vi "Last Ack Event.vi"(10 "Event":refnum<class "Event.lvclass">, 11 "Base Queue in":refnum<class "Base Queue.lvclass">) -> (3 "Base Queue out":refnum<class "Base Queue.lvclass">)   [LabVIEW 2021, in "jettl.lvlib" / "Base Queue.lvlib" / "Base Queue.lvclass"]
uses:
  Base Queue.lvclass
  Event/Event.lvclass
  Base Queue.lvclass/Base Queue.ctl
  Queue Mailbox/Queue Mailbox.lvlib
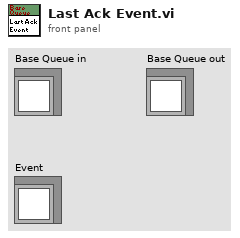
[diagram p1: front panel]
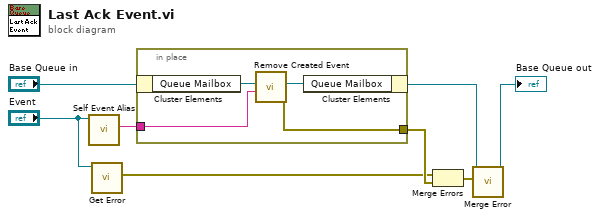
[diagram p0: block diagram]
diagram:
  n1 = call-dynamic "Self Event Alias.vi"("Event in"="Event") -> ("Self Event Alias"=w5:string)  [unwired: 10 in]
  n2 = call-dynamic "Get Error.vi"("jettl in"="Event") -> ("Error"=w1:errorcluster)  [unwired: 10 in]
  n3 = in-place {
    in-place-border: w5 -> [w11]
    in-place-border: [w9] -> w6
    n4 = in-place-cluster #1("Base Queue in") -> ("Queue Mailbox"=w12:refnum<data-value>)
    n5 = call "Remove Created Event.vi"("Self Event Alias"=w11, "Queue Mailbox in"=w12) -> ("error out"=w9:errorcluster, "Queue Mailbox out"=w10:refnum<data-value>)  [unwired: 8 in]
    n6 = in-place-cluster #1("Queue Mailbox"=w10) -> (w8:refnum<class "Base Queue.lvclass">)
  }
  n7 = Merge Errors(w1, w6) -> (w7:errorcluster)
  n8 = call-dynamic "Merge Error.vi"("Error"=w7, "Base Queue in"=w8) -> ("Base Queue out"=→"Base Queue out":refnum<class "Base Queue.lvclass">)  [unwired: 9 in]
